vi "Parser_0x53_(SubVI).vi"(11 "String in":string) -> (1 "кол-во считанных байт тела запрошенного параметра":i32, 2 "Начальное смещение в байтах":i32, 3 "Номер табличного параметра":i32)   [LabVIEW 2017, in "LV_Unicorn.lvlib"]
uses:
  LV_Unicorn.lvlib
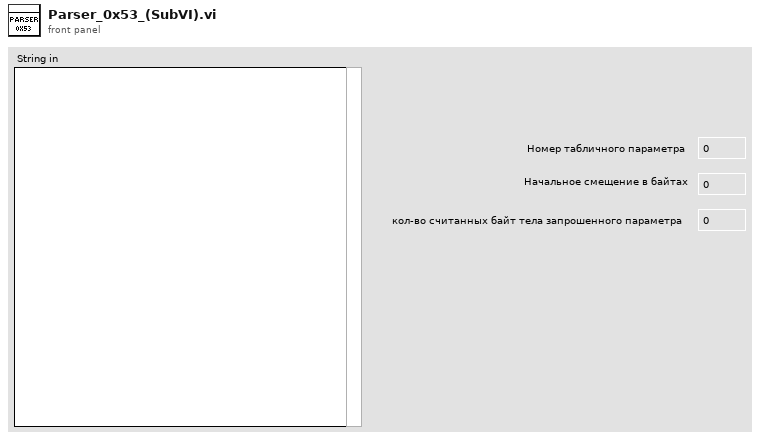
[diagram p1: front panel]
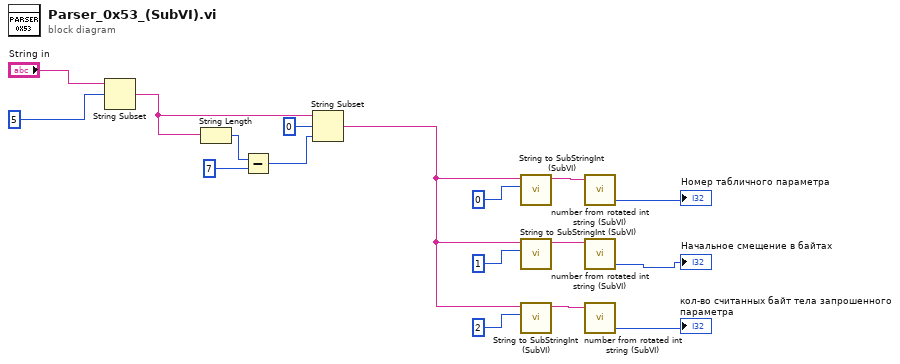
[diagram p0: block diagram]
diagram:
  n1 = String Subset(string="String in", offset (0)=5) -> (substring=w1:string)  [unwired: 1 in]
  n2 = String Length(string=w1) -> (length=w6:i32)
  n3 = Subtract(x=w6, y=7) -> (x-y=w2:i32)
  n4 = String Subset(string=w1, offset (0)=0, length (rest)=w2) -> (substring=w3:string)
  n5 = call "String to SubStringInt (SubVI).vi"("Nx4byte"=u32 0, "String in in"=w3) -> ("String out"=w10:string)  [unwired: 9 in]
  n6 = call "String to SubStringInt (SubVI).vi"("Nx4byte"=u32 1, "String in in"=w3) -> ("String out"=w11:string)  [unwired: 9 in]
  n7 = call "String to SubStringInt (SubVI).vi"("Nx4byte"=u32 2, "String in in"=w3) -> ("String out"=w15:string)  [unwired: 9 in]
  n8 = call "number from rotated int string (SubVI).vi"("String"=w10) -> ("int number"=→"Номер табличного параметра":i32)  [unwired: 2 in, 2 out]
  n9 = call "number from rotated int string (SubVI).vi"("String"=w11) -> ("int number"=→"Начальное смещение в байтах":i32)  [unwired: 2 in, 2 out]
  n10 = call "number from rotated int string (SubVI).vi"("String"=w15) -> ("int number"=→"кол-во считанных байт тела запрошенного параметра":i32)  [unwired: 2 in, 2 out]
